vi "pid2.v1.vi"() -> ()   [LabVIEW 2019]
doc: "The myRIO Project template acquires acceleration data from the onboard accelerometer and displays the changes of acceleration values in a waveform chart."
uses:
  <vilib>/addons/control/pid/NI_PID_pid.lvlib
  <vilib>/addons/control/pid/pid.llb/PID (DBL).vi
  <vilib>/ptbypt/NI_PtbyPt.lvlib
panel:
  out "servo":dbl
  out "output":dbl format="%.1f"
  out "Waveform Chart":cluster{"Setpoint":dbl, dbl, "servo":dbl}(graph)
  out "Winkel":dbl format="%.1g"
  out "Slide":dbl(slide) scale=0.0..60.0
  out "Sensor":dbl format="%0.2f"
  out "Waveform Graph":dbl[][](graph)
  out "Process Variable and Setpoint":cluster{dbl, dbl}(knob)={0.0, 10.0} scale=0.0..100.0
  in  "Output range":cluster{"output high":dbl, "output low":dbl}={"output high"=100.0, "output low"=-100.0} {"output low" format="%.3f"; "output high" format="%.3f"}
  in  "reinitialize? (F)":bool
  in  "PID gains":T1={"proportional gain (Kc)"=1.0, "integral time (Ti, min)"=0.01, "derivative time (Td, min)"=0.0} {"derivative time (Td, min)" format="%.3f"; "integral time (Ti, min)" format="%.3f"; "proportional gain (Kc)" format="%.3f"}
  in  "Setpoint":dbl(knob) scale=10.0..90.0
  in  "Stop":bool
  # "HC-SR04 ultrasonic module to measure distances in the range 2cm – 400cm."
  # "Connection:  Vcc to Pin 1 (Green + Black)   Port A"
  # "Gnd to Pin 12 (Green + Black) Port A"
  # "Trig to Pin 11 (Yellow) Port A"
  # "Echo to Pin 13 (Green) Port A"
  # "PWM to Pin 27 (Purple +Brown) Port A"
  # "Green Needle - PV"
  # "Red Needle - Setpoint"
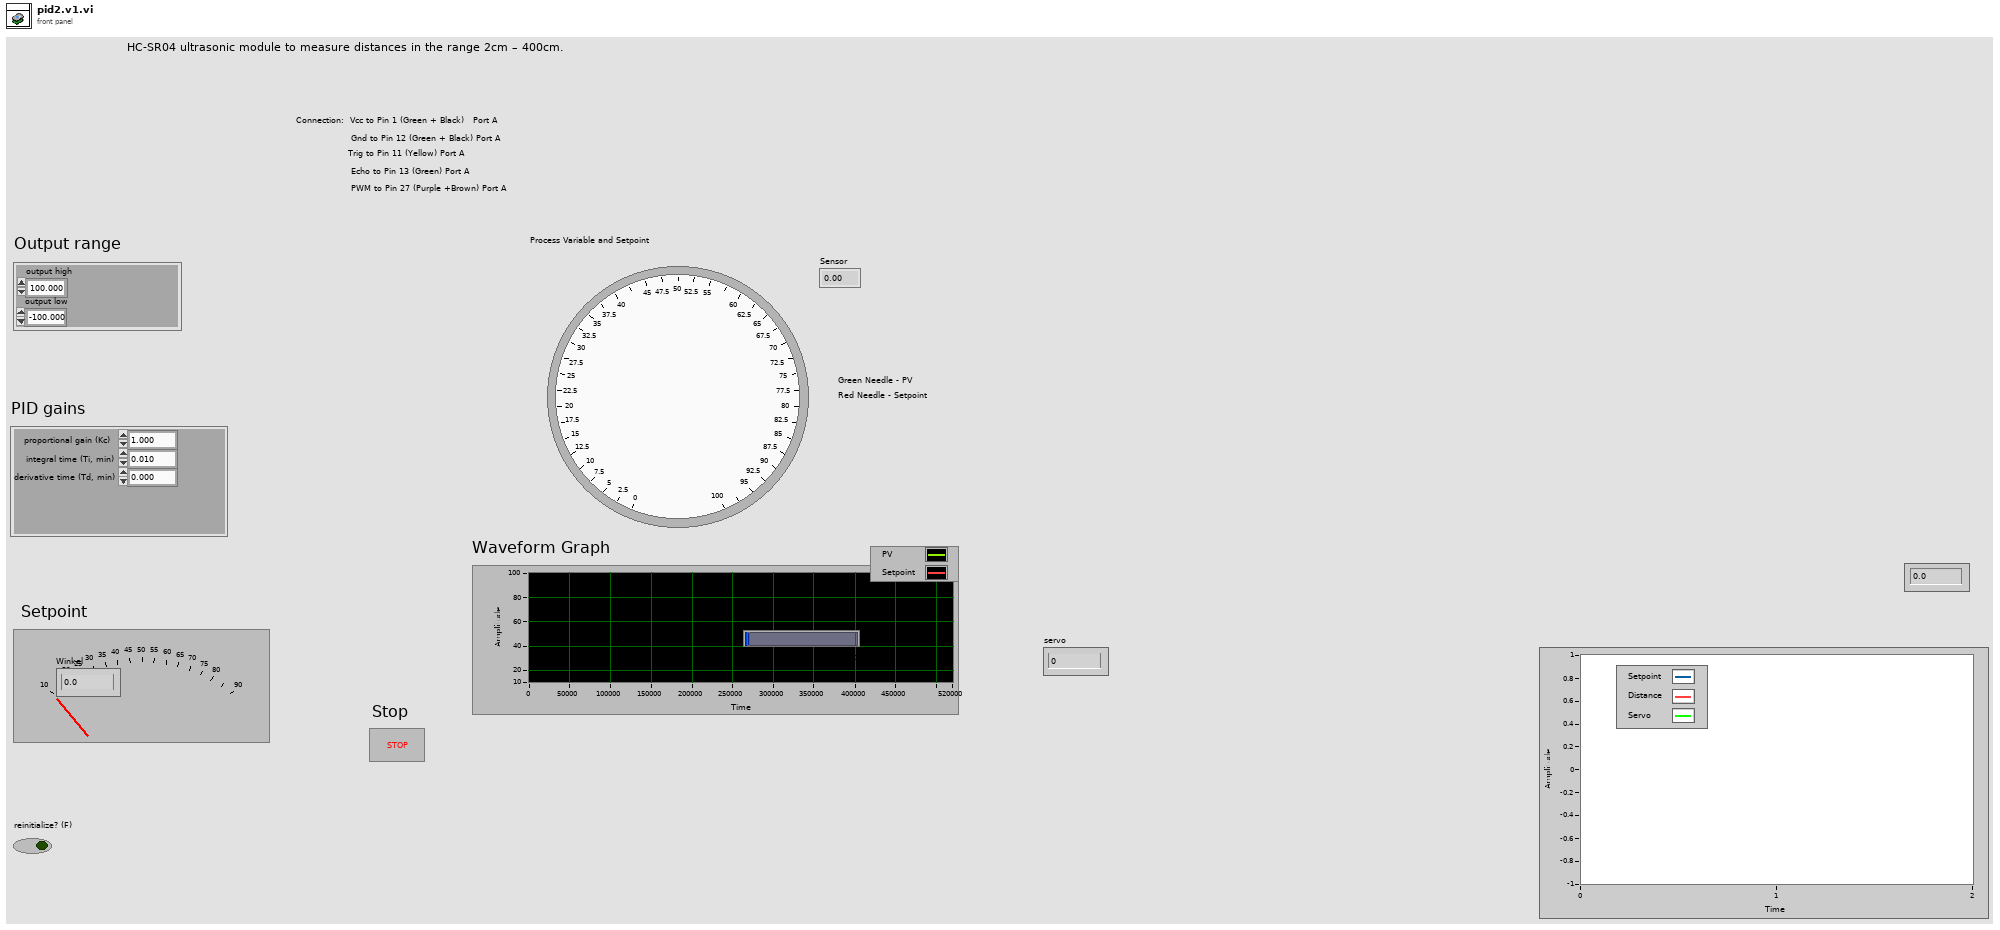
[diagram p1: front panel]
types:
  T1 = cluster{"proportional gain (Kc)":dbl, "integral time (Ti, min)":dbl, "derivative time (Td, min)":dbl}
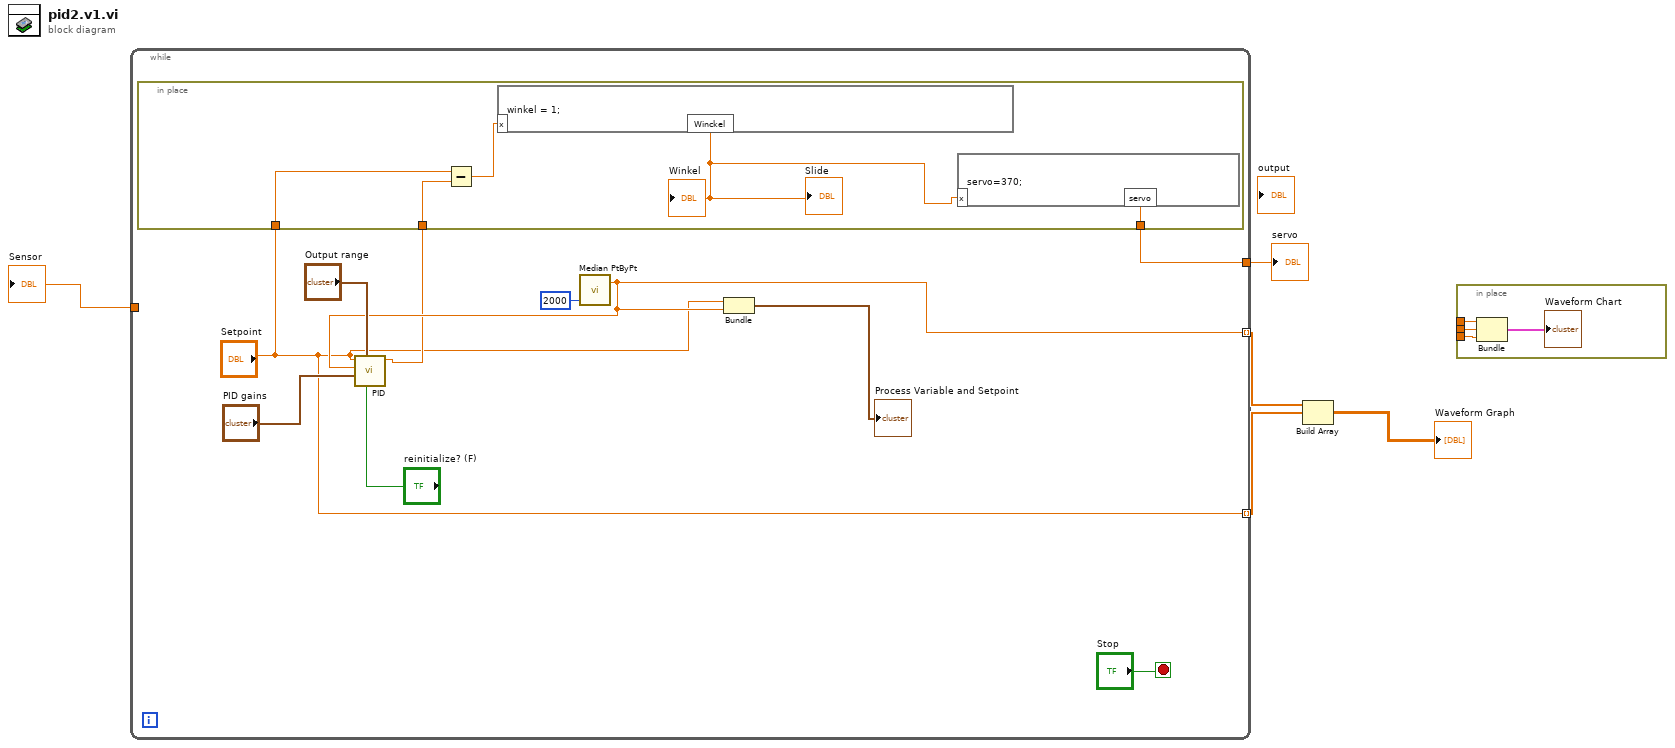
[diagram p0: block diagram]
diagram:
  n1 = while {
    tunnel: [w10] -> w5 mode=indexing
    tunnel: ["Setpoint"] -> w6 mode=indexing
    tunnel: [_] -> w3
    tunnel: [w7] -> w1
    stop <- "Stop" stop-if-true
    n2 = call <vilib>:"Median PtByPt.vi"("sample length"=2000) -> ("median"=w10:dbl)  [unwired: 3 in, 1 out]
    n3 = call-poly <vilib>:"PID.vi"("reinitialize? (F)"="reinitialize? (F)", "output range"="Output range", "PID gains"="PID gains", "process variable"=w10, "setpoint"="Setpoint") -> ("output"=w9:dbl)  [unwired: 5 in, 1 out]
    n4 = in-place {
      in-place-border: [w20] -> w7
      in-place-border: w9 -> [w18]
      in-place-border: "Setpoint" -> [w17]
      n5 = Subtract(x=w17, y=w18) -> (x-y=w19:dbl)
      n6 = formula code="winkel = 1;"("x"=w19) -> ("Winckel"=w21:dbl)
      "Winkel" <- w21
      "Slide" <- w21
      n7 = formula code="servo=370;"("x"=w21) -> ("servo"=w20:dbl)
    }
    n8 = Bundle("Setpoint"="Setpoint", "median"=w10) -> (→"Process Variable and Setpoint":cluster{"Setpoint":dbl, "median":dbl})  [unwired: 1 in]
  }
  "Sensor" <- w3
  "servo" <- w1
  n9 = Build Array(w5, w6) -> (→"Waveform Graph":dbl[][])  [unwired: 1 in]
  n10 = in-place {
    in-place-border: _ -> [w24]
    in-place-border: _ -> [w23]
    in-place-border: _ -> [w22]
    n11 = Bundle(w24, w23, w22) -> (→"Waveform Chart":cluster{void, void, void})  [unwired: 1 in]
  }
